vi "OCV DMM Clear Acquisition.vi"(8 "error in (no error)":errorcluster, 11 "Refnum in":refnum<k15>) -> (0 "error out":errorcluster, 4 "Clear Time (ms)":u32=46)   [LabVIEW 2019]
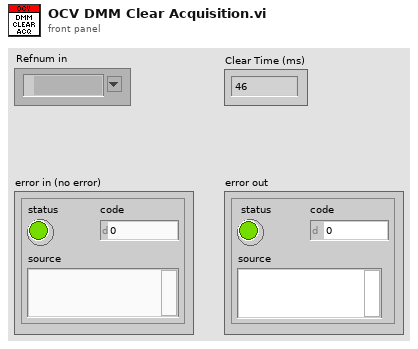
[diagram p1: front panel]
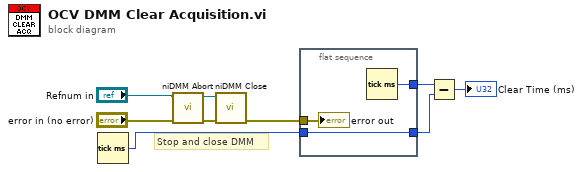
[diagram p0: block diagram]
diagram:
  # "Stop and close DMM"
  n1 = Tick Count (ms)() -> (millisecond timer value=w5:u32)
  n2 = call <instrlib>:"niDMM Abort.vi"("instrument handle"="Refnum in") -> ("error out"=w3:errorcluster, "instrument handle out"=w4:refnum<k15>)  [unwired: 9 in]
  n3 = call <instrlib>:"niDMM Close.vi"("error in (no error)"=w3, "instrument handle"=w4) -> ()  [unwired: 9 in, 1 out]
  n4 = flat-sequence {
    tunnel: "error in (no error)" -> [w10]
    tunnel: [w11] -> w6
    tunnel: w5 -> [w9]
    tunnel: [w9] -> w7
    frame #0 {
      n5 = Tick Count (ms)() -> (millisecond timer value=w11:u32)
      "error out" <- w10
    }
  }
  n6 = Subtract(x=w6, y=w7) -> (x-y=→"Clear Time (ms)":u32)
